vi "CreateHTML.vi"(0 "reference in":refnum<class "BooleanControl.lvclass">, 2 "VI Name":string, 5 "error in (no error)":errorcluster) -> (13 "script dependencies":string[](array[string]), 14 "reference out":refnum<class "BooleanControl.lvclass">, 15 "HTML":string, 16 "js variables":string, 17 "js code for controls":string, 18 "js code for indicators":string, 19 "error out":errorcluster)   [LabVIEW 2014, in "BooleanControl.lvclass"]
uses:
  BooleanControl.lvclass
  Text_class/Text.lvclass
  Object_class/Object.lvclass
  Control_class/Control.lvclass
  FrontPanelManager_class/FrontPanelManager.lvclass
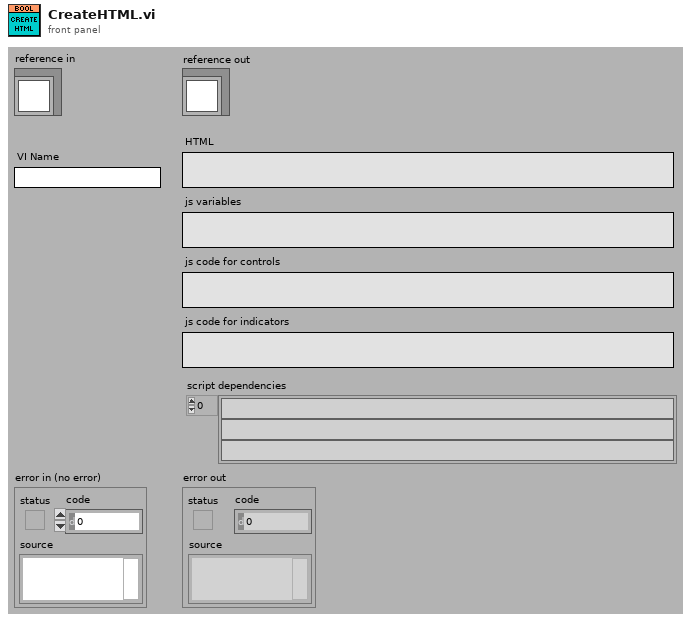
[diagram p1: front panel]
types:
  T1 = typedef "Object.lvclass/Attributes.ctl" = cluster{"UID":i32, "Type":string, "Coordinates":T2}
  T2 = typedef "Object.lvclass/Coordinates.ctl" = cluster{"Left":i32, "Top":i32, "Height":u32, "Width":u32}
  T3 = typedef "Control.lvclass/Attributes.ctl" = cluster{"Description":string, "Indicator":bool, "Default Value":variant, "Control Index":i32, "Label":refnum<class "Text.lvclass">, "Caption":refnum<class "Text.lvclass">, "Use Picture":bool, "Image 1":T4, "Image 2":T4}
  T4 = typedef "imagedata.ctl" = cluster{"image type":i32, "image depth":i32, "image":u8[], "mask":u8[], "colors":u32[], "Rectangle":cluster{"left":i16, "top":i16, "right":i16, "bottom":i16}}
  T5 = typedef "BooleanControl.lvclass/Attributes.ctl" = cluster{"Boolean ref":refnum<vi>, "Switching":bool, "Boolean Strings":string[], "Text":refnum<class "Text.lvclass">}
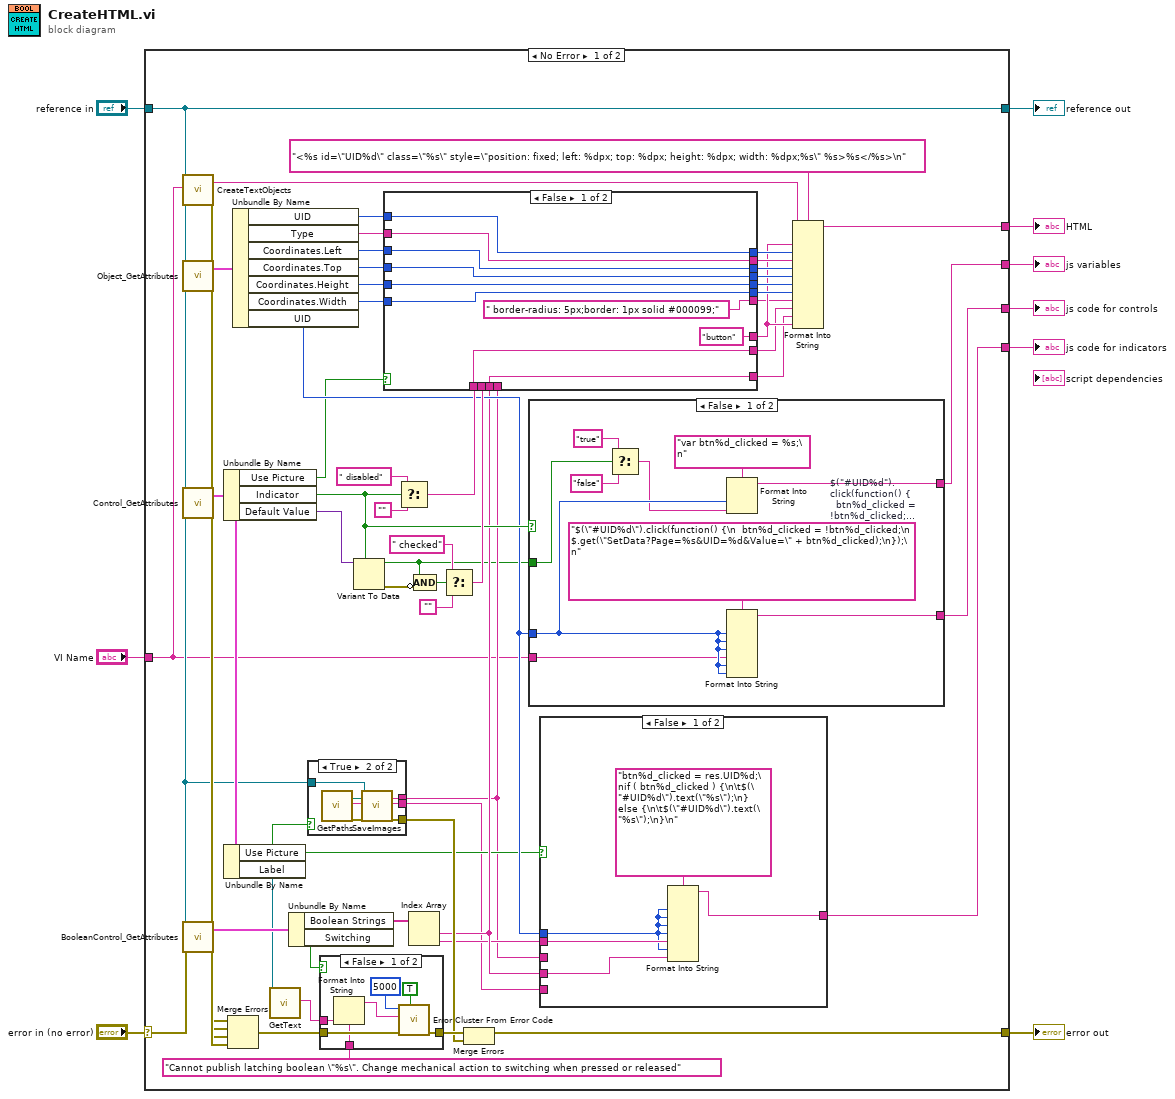
[diagram p0: block diagram]
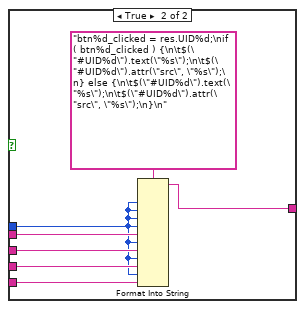
[diagram p4: hidden frame]
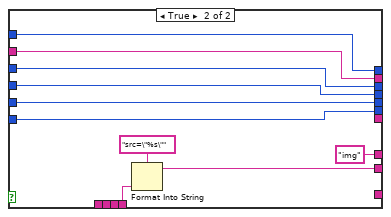
[diagram p6: hidden frame]
diagram:
  n1 = case shown="No Error" "error in (no error)" {
    selector: "error in (no error)" -> [w68 w127]
    tunnel: [w64 w127] -> w8
    tunnel: [w12 w126] -> w6
    tunnel: "reference in" -> [w12 w126]
    tunnel: [w57 _] -> w5
    tunnel: [w31 _] -> w4
    tunnel: [w30 _] -> w3
    tunnel: [w26 _] -> w2
    tunnel: "VI Name" -> [w11 _]
    frame No Error {
      n2 = call-dynamic "CreateTextObjects.vi"("reference in"=w12, "VI Name"=w11) -> ("HTML"=w10:string, "error out"=w59:errorcluster)  [unwired: 15 in, 1 out]
      n3 = call "Object_GetAttributes.vi"("reference in"=w12) -> ("Data"=w56:T1, "error out"=w60:errorcluster)  [unwired: 15 in, 2 out]
      n4 = call "Control_GetAttributes.vi"("reference in"=w12) -> ("Data"=w32:T3, "error out"=w61:errorcluster)  [unwired: 15 in, 2 out]
      n5 = call "BooleanControl_GetAttributes.vi"("reference in"=w12, "error in (no error)"=w68) -> ("Data"=w43:T5, "error out"=w65:errorcluster)  [unwired: 14 in, 2 out]
      n6 = Unbundle By Name(w32) -> ("Use Picture"=w23:bool, "Indicator"=w33:bool, "Default Value"=w36:variant)
      n7 = Unbundle By Name(w32) -> ("Use Picture"=w20:bool, "Label"=w16:refnum<class "Text.lvclass">)
      n8 = Merge Errors(w59, w60, w61, w65) -> (w62:errorcluster)
      n9 = Unbundle By Name(w56) -> ("UID"=w55:i32, "Type"=w54:string, "Coordinates.Left"=w53:i32, "Coordinates.Top"=w52:i32, "Coordinates.Height"=w51:u32, "Coordinates.Width"=w50:u32, "UID"=w27:i32)
      n10 = call-dynamic "GetText.vi"("reference in"=w16) -> ("Text"=w15:string)  [unwired: 16 in, 2 out]
      n11 = Unbundle By Name(w43) -> ("Boolean Strings"=w34:string[], "Switching"=w13:bool)
      n12 = case shown="True" w20 {
        tunnel: w12 -> [_ w79]
        tunnel: [_ w78] -> w18
        tunnel: [_ w77] -> w19
        tunnel: [_ w82] -> w63
        frame False {
        }
        frame True {
          n13 = call "GetPaths.vi"() -> ("Image folder"=w80:path, "Image URL"=w81:string, "error out"=w83:errorcluster)  [unwired: 16 in, 1 out]
          n14 = call-dynamic "SaveImages.vi"("reference in"=w79, "Image path"=w80, "Image URL"=w81, "error in (no error)"=w83) -> ("Image 1 URL"=w78:string, "Image 2 URL"=w77:string, "error out"=w82:errorcluster)  [unwired: 12 in, 1 out]
        }
      }
      n15 = case shown="False" w13 {
        tunnel: [w75 w76] -> w66
        tunnel: w62 -> [w74 w76]
        tunnel: w15 -> [w71 _]
        tunnel: "Cannot publish latching boolean \"%s\". Change mechanical action to switching when pressed or released" -> [w70 _]
        frame False {
          n16 = Format Into String(format string=w70, w71) -> (resulting string=w69:string)  [unwired: 2 in, 1 out]
          n17 = call <vilib>:"Error Cluster From Error Code.vi"("show call chain? (False)"=TRUE, "error in (no error)"=w74, "error message (\"\")"=w69, "error code (0)"=5000) -> ("error out"=w75:errorcluster)  [unwired: 5 in]
        }
        frame True {
        }
      }
      n18 = Variant To Data(type=w33, Variant=w36) -> (data=w17:bool, error out=w67:errorcluster)  [unwired: 1 in]
      n19 = Select(t=" disabled", s=w33, f="") -> (s? t:f=w40:string)
      n20 = Index Array(array=w34) -> (element #1=w25:string, element #2=w24:string)  [unwired: 2 in]
      n21 = Compound Arithmetic op=AND(w17, invert w67) -> (w39:bool)
      n22 = Select(t=" checked", s=w39, f="") -> (s? t:f=w35:string)
      n23 = case shown="False" w23 {
        tunnel: ["button" "img"] -> w29
        tunnel: w40 -> [w106 _]
        tunnel: w35 -> [_ _]
        tunnel: [w114 _] -> w28
        tunnel: w25 -> [w114 _]
        tunnel: [w106 w116] -> w21
        tunnel: [w112 w124] -> w48
        tunnel: w54 -> [w112 w124]
        tunnel: [w113 w123] -> w49
        tunnel: w55 -> [w113 w123]
        tunnel: [w111 w122] -> w47
        tunnel: w53 -> [w111 w122]
        tunnel: [w110 w121] -> w46
        tunnel: w52 -> [w110 w121]
        tunnel: [w108 w120] -> w44
        tunnel: w50 -> [w108 w120]
        tunnel: w51 -> [w109 w119]
        tunnel: [w109 w119] -> w45
        tunnel: [" border-radius: 5px;border: 1px solid #000099;" _] -> w22
        tunnel: w18 -> [_ w117]
        frame False {
        }
        frame True {
          n24 = Format Into String(format string="src=\"%s\"", w117) -> (resulting string=w116:string)  [unwired: 2 in, 1 out]
        }
      }
      n25 = Merge Errors(w66, w63) -> (w64:errorcluster)
      n26 = case shown="False" w33 {
        tunnel: [w105 _] -> w30
        tunnel: w27 -> [w104 _]
        tunnel: [w103 _] -> w31
        tunnel: w11 -> [w102 _]
        tunnel: w17 -> [w99 _]
        frame False {
          w101 = "$(\"#UID%d\").click(function() {\n  btn%d_clicked = !btn%d_clicked;\n  $.get(\"SetData?Page=%s&UID=%d&Value=\" + btn%d_clicked);\n});\n"  # $("#UID%d").click(function() {   btn%d_clicked = !btn%d_clicked;   $.get("SetData?Page=%s&UID=%d&Value=" + btn%d_clicked); });
          n27 = Select(t="true", s=w99, f="false") -> (s? t:f=w96:string)
          n28 = Format Into String(format string="var btn%d_clicked = %s;\n", w104, w96) -> (resulting string=w103:string)  [unwired: 2 in, 1 out]
          n29 = Format Into String(format string=w101, w104, w104, w104, w102, w104, w104) -> (resulting string=w105:string)  [unwired: 2 in, 1 out]
        }
        frame True {
        }
      }
      n30 = case shown="False" w20 {
        tunnel: w24 -> [w88 w95]
        tunnel: w27 -> [w84 w89]
        tunnel: [w87 w94] -> w26
        tunnel: w25 -> [w85 w92]
        tunnel: w18 -> [_ w91]
        tunnel: w19 -> [_ w90]
        frame False {
          n31 = Format Into String(format string="btn%d_clicked = res.UID%d;\nif ( btn%d_clicked ) {\n\t$(\"#UID%d\").text(\"%s\");\n} else {\n\t$(\"#UID%d\").text(\"%s\");\n}\n", w84, w84, w84, w84, w88, w84, w85) -> (resulting string=w87:string)  [unwired: 2 in, 1 out]
        }
        frame True {
          n32 = Format Into String(format string="btn%d_clicked = res.UID%d;\nif ( btn%d_clicked ) {\n\t$(\"#UID%d\").text(\"%s\");\n\t$(\"#UID%d\").attr(\"src\", \"%s\");\n} else {\n\t$(\"#UID%d\").text(\"%s\");\n\t$(\"#UID%d\").attr(\"src\", \"%s\");\n}\n", w89, w89, w89, w89, w95, w89, w91, w89, w92, w89, w90) -> (resulting string=w94:string)  [unwired: 2 in, 1 out]
        }
      }
      n33 = Format Into String(format string="<%s id=\"UID%d\" class=\"%s\" style=\"position: fixed; left: %dpx; top: %dpx; height: %dpx; width: %dpx;%s\" %s>%s</%s>\n", initial string=w10, w29, w49, w48, w47, w46, w45, w44, w22, w21, w28, w29) -> (resulting string=w57:string)  [unwired: 1 in, 1 out]
    }
    frame Error {
    }
  }
  "error out" <- w8
  "reference out" <- w6
  "HTML" <- w5
  "js variables" <- w4
  "js code for controls" <- w3
  "js code for indicators" <- w2
